vi "hexToStr.vi"(1 "strType":enum16{"normal", "Hex"}(ring)=enum."Hex", 5 "str":string) -> (6 "strOut":string)   [LabVIEW 2015]
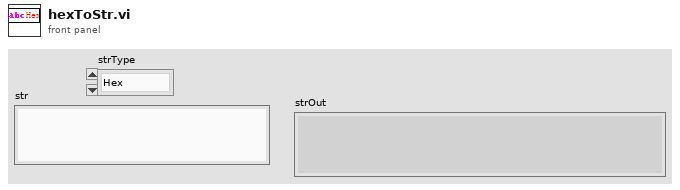
[diagram p1: front panel]
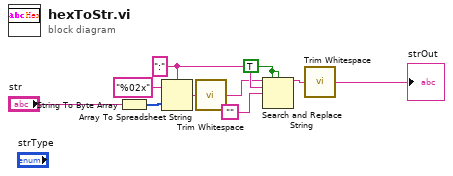
[diagram p0: block diagram]
diagram:
  w3 = TRUE ("忽略大小写？(F)")
  w7 = ":" ("分隔符(Tab)")
  n1 = String To Byte Array(string="str") -> (unsigned byte array=w10:u8[])
  n2 = Array To Spreadsheet String(delimiter (Tab)=w7, array=w10, 3:"%02x" ("格式字符串")) -> (spreadsheet string=w8:string)
  n3 = call <vilib>:"Trim Whitespace.vi"("string"=w8) -> ("trimmed string"=w4:string)  [unwired: 1 in]
  n4 = Search and Replace String(replace all?=w3, case sensitive?=w3, input string=w4, search string=w7, replace string="") -> (result string=w5:string)  [unwired: 3 in, 3 out]
  n5 = call <vilib>:"Trim Whitespace.vi"("string"=w5) -> ("trimmed string"=→"strOut":string)  [unwired: 1 in]
